vi "Create CircularBuffer ByType.vi"(5 "Buffer Name":string, 7 "CircularBuffer in":refnum<class "CircularBuffer.lvclass">, 8 "error in (no error)":errorcluster, 9 "type":refnum<class "type.lvclass">, 11 "BufferSize":i32=1) -> (0 "error out":errorcluster, 2 "Buffer name created":string, 3 "CircularBuffer out":refnum<class "CircularBuffer.lvclass">)   [LabVIEW 2013, in "CircularBuffer.lvclass"]
uses:
  CircularBuffer.lvclass
  <vilib>/JKI/JKI SMO/SMO/SMO.lvclass
  types/type/type.lvclass
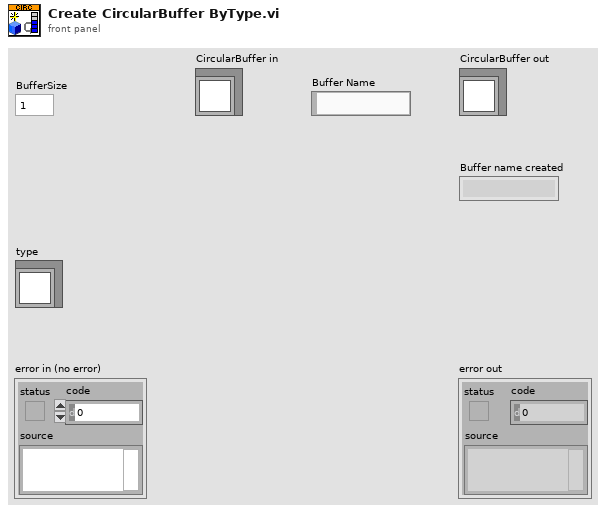
[diagram p1: front panel]
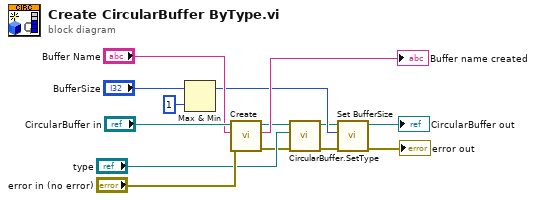
[diagram p0: block diagram]
diagram:
  n1 = Max & Min(x="BufferSize", y=1) -> (max(x,y)=w9:i32)  [unwired: 1 out]
  n2 = call <vilib>:"Create.vi"("error in (no error)"="error in (no error)", "Subsystem Name (optional)"="Buffer Name", "SMO"="CircularBuffer in") -> ("error out"=w4:errorcluster, "SMO name"=→"Buffer name created":string, "SMO out"=w6:refnum<class "CircularBuffer.lvclass">)  [unwired: 6 in]
  n3 = call "CircularBuffer.SetType.vi"("error in (no error)"=w4, "type"="type", "CircularBuffer"=w6) -> ("error out"=w3:errorcluster, "CircularBuffer out"=w5:refnum<class "CircularBuffer.lvclass">)  [unwired: 7 in]
  n4 = call "Set BufferSize.vi"("error in (no error)"=w3, "Buffer Size"=w9, "CircularBuffer"=w5) -> ("error out"=→"error out":errorcluster, "CircularBuffer out"=→"CircularBuffer out":refnum<class "CircularBuffer.lvclass">)  [unwired: 7 in]
